vi "Set Detection.vi"(8 "error in (no error)":errorcluster, 10 "Detection":T1, 11 "Ti2 in":refnum<class "Ti2.lvclass">) -> (0 "error out":errorcluster, 3 "Ti2 out":refnum<class "Ti2.lvclass">)   [LabVIEW 2018, in "Ti2.lvlib" / "Ti2.lvclass"]
uses:
  Ti2.lvclass
  ti2lv/ti2lv.lvlib
  ti2lv/ti2_lightPath.ctl
  ti2lv/ti2_filterPos.ctl
  Resources/Type Defs/Detection.ctl
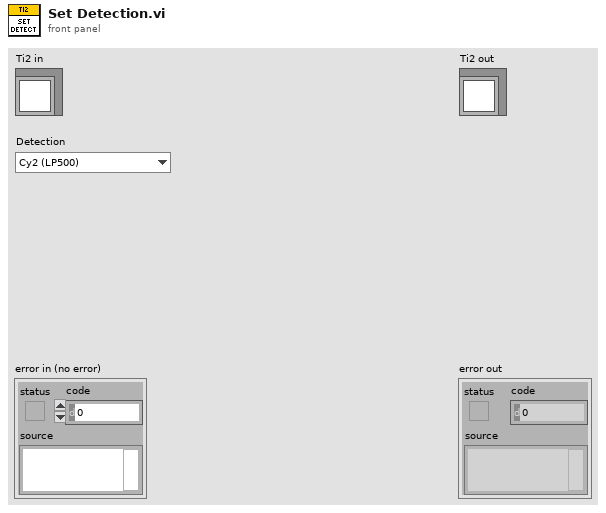
[diagram p1: front panel]
types:
  T1 = typedef "Detection.ctl" = enum16{"Cy2 (LP500)", "Cy3 (LP550)", "Cy5 (BP700/75)", "Cy3/Cy5 (BP590/40,700/60)", "No Filter", "Laser to Eyes"}
  T2 = typedef "ti2lv.lvlib/ti2_lightPath.ctl" = i32
  T3 = typedef "ti2lv.lvlib/ti2_filterPos.ctl" = u16
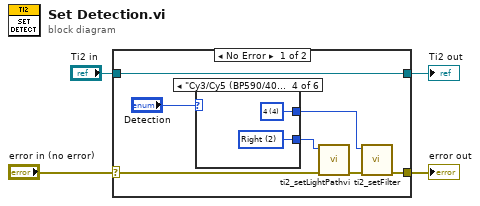
[diagram p0: block diagram]
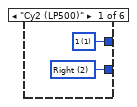
[diagram p2: hidden frame]
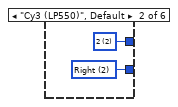
[diagram p3: hidden frame]
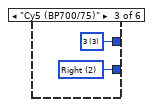
[diagram p4: hidden frame]
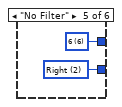
[diagram p5: hidden frame]
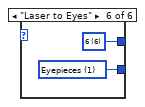
[diagram p6: hidden frame]
diagram:
  n1 = case shown="No Error" "error in (no error)" {
    selector: "error in (no error)" -> [w7 w25]
    tunnel: [w5 w25] -> w3
    tunnel: [w11 w24] -> w1
    tunnel: "Ti2 in" -> [w11 w24]
    frame No Error {
      n2 = case shown="\"Cy3/Cy5 (BP590/40,700/60)\"" "Detection" {
        tunnel: [w12 w14 w16 w18 w20 w23] -> w8
        tunnel: [w13 w15 w17 w19 w21 w22] -> w9
        frame "Cy2 (LP500)" {
          w12 = T2 2 items=["Eyepieces"=1, "Right"=2, "Bottom"=3, "Left"=4] ("Light Path")
          w13 = T3 1 items=["1"=1, "2"=2, "3"=3, "4"=4, "5"=5, "6"=6] ("Filter Position")
        }
        frame "Cy3 (LP550)", Default {
          w14 = T2 2 items=["Eyepieces"=1, "Right"=2, "Bottom"=3, "Left"=4] ("Light Path")
          w15 = T3 2 items=["1"=1, "2"=2, "3"=3, "4"=4, "5"=5, "6"=6] ("Filter Position")
        }
        frame "Cy5 (BP700/75)" {
          w16 = T2 2 items=["Eyepieces"=1, "Right"=2, "Bottom"=3, "Left"=4] ("Light Path")
          w17 = T3 3 items=["1"=1, "2"=2, "3"=3, "4"=4, "5"=5, "6"=6] ("Filter Position")
        }
        frame "Cy3/Cy5 (BP590/40,700/60)" {
          w18 = T2 2 items=["Eyepieces"=1, "Right"=2, "Bottom"=3, "Left"=4] ("Light Path")
          w19 = T3 4 items=["1"=1, "2"=2, "3"=3, "4"=4, "5"=5, "6"=6] ("Filter Position")
        }
        frame "No Filter" {
          w20 = T2 2 items=["Eyepieces"=1, "Right"=2, "Bottom"=3, "Left"=4] ("Light Path")
          w21 = T3 6 items=["1"=1, "2"=2, "3"=3, "4"=4, "5"=5, "6"=6] ("Filter Position")
        }
        frame "Laser to Eyes" {
          w22 = T3 6 items=["1"=1, "2"=2, "3"=3, "4"=4, "5"=5, "6"=6] ("Filter Position")
          w23 = T2 1 items=["Eyepieces"=1, "Right"=2, "Bottom"=3, "Left"=4] ("Light Path")
        }
      }
      n3 = call "ti2_setLightPathvi.vi"("error in (no error)"=w7, "Light Path"=w8) -> ("error out"=w6:errorcluster)  [unwired: 9 in]
      n4 = call "ti2_setFilter.vi"("error in (no error)"=w6, "Filter Position"=w9) -> ("error out"=w5:errorcluster)  [unwired: 9 in]
    }
    frame Error {
    }
  }
  "error out" <- w3
  "Ti2 out" <- w1
